vi "HFRR ADV v01.vi"() -> ()   [LabVIEW 2025] (continued)
            n3072 = case shown="True" w3184 {
              frame False {
              }
              frame True {
                n3073 = local write "Rt 3"(FALSE ("Rt 3")) -> ()
              }
            }
            "Rt" <- TRUE ("Rt")
            "Rt 2" <- FALSE ("Rt")
          }
          frame True {
            n3074 = local read "Rt"() -> (w3190:bool)
            n3075 = local write "Rt 2"(TRUE ("Rt 2")) -> ()
            n3076 = case shown="True" w3190 {
              frame False {
              }
              frame True {
                n3077 = local write "Rt"(FALSE ("Rt")) -> ()
              }
            }
            "Rt 3" <- TRUE ("Rt 3")
          }
        }
        n3078 = local read "Reset Graph"() -> (w3109:bool)
        n3079 = case shown="True" w3109 {
          selector: w3109 -> [_ w3133]
          frame False {
          }
          frame True {
            w3147 = 0.0 ("X Scale.Range:Maximum")
            n3080 = Not(x=w3133) -> (.not. x?=w3132:bool)
            n3081 = local write "Reset Graph"(w3132) -> ()
            n3082 = property on="Electrical Contact Resistance ( % )" class="WFChart (strict)"("XScale.Maximum"=600.0 ("X Scale.Range:Maximum"), "XScale.Minimum"=0.0 ("X Scale.Range:Minimum"), "YScale.Maximum"=100.0 ("Y Scale.Range:Maximum"), "YScale.Minimum"=0.0 ("Y Scale.Range:Minimum")) -> ()  [unwired: 2 in, 2 out]
            n3083 = property on="Frictional Force ( N )" class="WFChart (strict)"("XScale.Maximum"=600.0 ("X Scale.Range:Maximum"), "XScale.Minimum"=0.0 ("X Scale.Range:Minimum"), "YScale.Maximum"=100.0 ("Y Scale.Range:Maximum"), "YScale.Minimum"=0.0 ("Y Scale.Range:Minimum")) -> ()  [unwired: 2 in, 2 out]
            n3084 = property on="Temperature ( Deg C )" class="WFChart (strict)"("XScale.Maximum"=600.0 ("X Scale.Range:Maximum"), "XScale.Minimum"=0.0 ("X Scale.Range:Minimum"), "YScale.Maximum"=100.0 ("Y Scale.Range:Maximum"), "YScale.Minimum"=0.0 ("Y Scale.Range:Minimum")) -> ()  [unwired: 2 in, 2 out]
            n3085 = property on="Stroke ( mm )" class="WFChart (strict)"("XScale.Maximum"=600.0 ("X Scale.Range:Maximum"), "XScale.Minimum"=0.0 ("X Scale.Range:Minimum"), "YScale.Maximum"=100.0 ("Y Scale.Range:Maximum"), "YScale.Minimum"=0.0 ("Y Scale.Range:Minimum")) -> ()  [unwired: 2 in, 2 out]
            n3086 = property on="Coefficient of Friction" class="WFChart (strict)"("XScale.Maximum"=600.0 ("X Scale.Range:Maximum"), "XScale.Minimum"=0.0 ("X Scale.Range:Minimum"), "YScale.Maximum"=100.0 ("Y Scale.Range:Maximum"), "YScale.Minimum"=0.0 ("Y Scale.Range:Minimum")) -> ()  [unwired: 2 in, 2 out]
            n3087 = property on="Electrical Contact Resistance ( % )" class="WFChart (strict)"("XScale.Minimum"=0.0 ("X Scale.Range:Minimum"), "XScale.Maximum"=600.0 ("X Scale.Range:Maximum"), "YScale.Minimum"=0.0 ("Y Scale.Range:Minimum"), "YScale.Maximum"=100.0 ("Y Scale.Range:Maximum")) -> ()  [unwired: 2 in, 2 out]
            n3088 = property on="Temperature ( Deg C )" class="WFChart (strict)"("XScale.Minimum"=0.0 ("X Scale.Range:Minimum"), "XScale.Maximum"=600.0 ("X Scale.Range:Maximum"), "YScale.Minimum"=0.0 ("Y Scale.Range:Minimum"), "YScale.Maximum"=100.0 ("Y Scale.Range:Maximum")) -> ()  [unwired: 2 in, 2 out]
            n3089 = property on="Coefficient of Friction" class="WFChart (strict)"("XScale.Minimum"=0.0 ("X Scale.Range:Minimum"), "XScale.Maximum"=600.0 ("X Scale.Range:Maximum"), "YScale.Maximum"=1.0 ("X Scale.Range:Minimum"), "YScale.Minimum"=0.0 ("X Scale.Range:Minimum")) -> ()  [unwired: 2 in, 2 out]
            n3090 = property on="Frictional Force ( N )" class="WFChart (strict)"("XScale.Maximum"=600.0 ("X Scale.Range:Maximum"), "XScale.Minimum"=w3147, "YScale.Maximum"=10.0 ("Y Scale.Range:Maximum"), "YScale.Minimum"=w3147) -> ()  [unwired: 2 in, 2 out]
            n3091 = property on="Stroke ( mm )" class="WFChart (strict)"("XScale.Maximum"=600.0 ("X Scale.Range:Maximum"), "XScale.Minimum"=0.0 ("X Scale.Range:Minimum"), "YScale.Maximum"=100.0 ("Y Scale.Range:Maximum"), "YScale.Minimum"=0.0 ("Y Scale.Range:Minimum")) -> ()  [unwired: 2 in, 2 out]
          }
        }
      }
      frame "Compare Files" {
        # "Elapsed time\ncof\nstroke\nAir temp\nTemp\nHumidity"
        n3092 = case shown="True" "RSTV1 2" {
          frame False {
          }
          frame True {
            n3093 = property on="Humidity ( %RH )" class="XYGraph (strict)"("Y Scale.Display Format:Precision"=u8 0 ("Y Scale.Format & Precision:Precision")) -> ()  [unwired: 2 in, 2 out]
            n3094 = property on="Humidity ( %RH )" class="XYGraph (strict)"("X Scale.Range:Minimum"=0.0, "X Scale.Range:Maximum"=75.0, "Y Scale.Range:Minimum"=48.0, "Y Scale.Range:Maximum"=58.0) -> ()  [unwired: 2 in, 2 out]
          }
        }
        n3095 = case shown="True" "RST CP 2" {
          frame False {
          }
          frame True {
            n3096 = property on="XY Graph 13" class="XYGraph (strict)"("Y Scale.Display Format:Precision"=u8 0 ("Y Scale.Format & Precision:Precision")) -> ()  [unwired: 2 in, 2 out]
            n3097 = property on="XY Graph 13" class="XYGraph (strict)"("X Scale.Range:Minimum"=0.0, "X Scale.Range:Maximum"=75.0, "Y Scale.Range:Minimum"=0.0, "Y Scale.Range:Maximum"=100.0) -> ()  [unwired: 2 in, 2 out]
          }
        }
        n3098 = case shown="True" "RST CP" {
          frame False {
          }
          frame True {
            n3099 = property on="Sample Temperature ( °C )" class="XYGraph (strict)"("Y Scale.Display Format:Precision"=u8 2 ("Y Scale.Format & Precision:Precision")) -> ()  [unwired: 2 in, 2 out]
            n3100 = property on="Sample Temperature ( °C )" class="XYGraph (strict)"("X Scale.Range:Minimum"=0.0, "X Scale.Range:Maximum"=75.0, "Y Scale.Range:Minimum"=58.0, "Y Scale.Range:Maximum"=62.0) -> ()  [unwired: 2 in, 2 out]
          }
        }
        n3101 = case shown="True" "RSTV1 3" {
          frame False {
          }
          frame True {
            n3102 = property on="Air Temperature  ( °C )" class="XYGraph (strict)"("Y Scale.Display Format:Precision"=u8 2 ("Y Scale.Format & Precision:Precision")) -> ()  [unwired: 2 in, 2 out]
            n3103 = property on="Air Temperature  ( °C )" class="XYGraph (strict)"("X Scale.Range:Minimum"=0.0 ("Y Scale.Range:Minimum"), "X Scale.Range:Maximum"=75.0 ("Y Scale.Range:Maximum"), "Y Scale.Range:Minimum"=20.0 ("X Scale.Range:Minimum"), "Y Scale.Range:Maximum"=26.0 ("X Scale.Range:Maximum")) -> ()  [unwired: 2 in, 2 out]
          }
        }
        n3104 = case shown="True" "RSTV1 4" {
          frame False {
          }
          frame True {
            n3105 = property on="Stroke ( mm )" class="XYGraph (strict)"("Y Scale.Display Format:Precision"=u8 2 ("Y Scale.Format & Precision:Precision")) -> ()  [unwired: 2 in, 2 out]
            n3106 = property on="Stroke ( mm )" class="XYGraph (strict)"("X Scale.Range:Minimum"=0.0 ("Y Scale.Range:Maximum"), "X Scale.Range:Maximum"=75.0 ("X Scale.Range:Minimum"), "Y Scale.Range:Minimum"=0.98, "Y Scale.Range:Maximum"=1.02) -> ()  [unwired: 2 in, 2 out]
          }
        }
        n3107 = case shown="True" "rstv2" {
          frame False {
          }
          frame True {
            n3108 = property on="Coefficient Of Friction" class="XYGraph (strict)"("Y Scale.Display Format:Precision"=u8 3 ("Y Scale.Format & Precision:Precision")) -> ()  [unwired: 2 in, 2 out]
            n3109 = property on="Coefficient Of Friction" class="XYGraph (strict)"("X Scale.Range:Minimum"=0.0 ("Y Scale.Range:Maximum"), "X Scale.Range:Maximum"=75.0, "Y Scale.Range:Minimum"=0.0, "Y Scale.Range:Maximum"=1.0 ("X Scale.Range:Minimum")) -> ()  [unwired: 2 in, 2 out]
          }
        }
        n3110 = case shown="True" "RST CP 3" {
          frame False {
          }
          frame True {
            n3111 = property on="Air Temp ( °C ) vs Humidity ( % RH )" class="XYGraph (strict)"("X Scale.Range:Minimum"=18.0, "X Scale.Range:Maximum"=28.0 ("X Scale.Range:Minimum"), "Y Scale.Range:Minimum"=30.0 ("X Scale.Range:Minimum"), "Y Scale.Range:Maximum"=70.0 ("X Scale.Range:Minimum")) -> ()  [unwired: 2 in, 2 out]
          }
        }
        n3112 = case shown="True" "OPEN 1" {
          frame False {
          }
          frame True {
            (unwired) 0  # existing file
            w3900 = "Choose a datalog file to open"  # prompt
            n3113 = local write "OPEN 1"(FALSE ("OPEN 1")) -> ()
            n3114 = String To Path(string="C:\\LAB-IQ\\Data\\") -> (path=w3885:path)
            n3115 = File Dialog(6:"*.dgf" ("pattern"), 7:w3900, 11:w3885) -> (0:w3883:errorcluster, 3:w3891:path)  [unwired: 4 in, 2 out]
            n3116 = Unbundle(w3883) -> ()  [unwired: 3 out]
            n3117 = Strip Path(path=w3891) -> (name=w3890:string)  [unwired: 1 out]
            n3118 = Path To String(path=w3891) -> (string=w3886:string)
            "string1" <- w3886
            n3119 = Match Pattern(string=w3890, regular expression=".dgf") -> (before substring=→"String Control":string)  [unwired: 1 in, 3 out]
            n3120 = Match Pattern(string=w3886, regular expression=".dgf" ("substring (\"\")")) -> (before substring=w3896:string)  [unwired: 1 in, 3 out]
            n3121 = Concatenate Strings(w3896, ".duf" ("Substring")) -> (w3892:string)
            n3122 = String To Path(string=w3892) -> (path=w3897:path)
            n3123 = call <vilib>:"Read Characters From File.vi"("file path (dialog if empty)"=w3897, "start of read offset (chars.:0)"=60 ("start of read offset (chars.: 0)")) -> ("character string"=→"String Control 2":string)  [unwired: 4 in, 3 out]
          }
        }
        n3124 = case shown="True" "OPEN 2" {
          frame False {
          }
          frame True {
            (unwired) 0  # existing file
            w3918 = "Choose a datalog file to open"  # prompt
            n3125 = local write "OPEN 2"(FALSE ("OPEN 1")) -> ()
            n3126 = String To Path(string="C:\\LAB-IQ\\Data\\") -> (path=w3903:path)
            n3127 = File Dialog(6:"*.dgf" ("pattern"), 7:w3918, 11:w3903) -> (0:w3901:errorcluster, 3:w3909:path)  [unwired: 4 in, 2 out]
            n3128 = Unbundle(w3901) -> ()  [unwired: 3 out]
            n3129 = Strip Path(path=w3909) -> (name=w3907:string)  [unwired: 1 out]
            n3130 = Path To String(path=w3909) -> (string=w3904:string)
            "string1 2" <- w3904
            n3131 = Match Pattern(string=w3907, regular expression=".dgf") -> (before substring=→"String Control 3":string)  [unwired: 1 in, 3 out]
            n3132 = Match Pattern(string=w3904, regular expression=".dgf" ("substring (\"\")")) -> (before substring=w3915:string)  [unwired: 1 in, 3 out]
            n3133 = Concatenate Strings(w3915, ".duf" ("Substring")) -> (w3912:string)
            n3134 = String To Path(string=w3912) -> (path=w3910:path)
            n3135 = call <vilib>:"Read Characters From File.vi"("file path (dialog if empty)"=w3910, "start of read offset (chars.:0)"=60 ("start of read offset (chars.: 0)")) -> ("character string"=→"String Control 4":string)  [unwired: 4 in, 3 out]
          }
        }
        n3136 = case shown="True" "OPEN 3" {
          frame False {
          }
          frame True {
            (unwired) 0  # existing file
            w3936 = "Choose a datalog file to open"  # prompt
            n3137 = local write "OPEN 3"(FALSE ("OPEN 1")) -> ()
            n3138 = String To Path(string="C:\\LAB-IQ\\Data\\") -> (path=w3921:path)
            n3139 = File Dialog(6:"*.dgf" ("pattern"), 7:w3936, 11:w3921) -> (0:w3919:errorcluster, 3:w3927:path)  [unwired: 4 in, 2 out]
            n3140 = Unbundle(w3919) -> ()  [unwired: 3 out]
            n3141 = Strip Path(path=w3927) -> (name=w3925:string)  [unwired: 1 out]
            n3142 = Path To String(path=w3927) -> (string=w3922:string)
            "string1 3" <- w3922
            n3143 = Match Pattern(string=w3925, regular expression=".dgf") -> (before substring=→"String Control 5":string)  [unwired: 1 in, 3 out]
            n3144 = Match Pattern(string=w3922, regular expression=".dgf" ("substring (\"\")")) -> (before substring=w3932:string)  [unwired: 1 in, 3 out]
            n3145 = Concatenate Strings(w3932, ".duf" ("Substring")) -> (w3929:string)
            n3146 = String To Path(string=w3929) -> (path=w3933:path)
            n3147 = call <vilib>:"Read Characters From File.vi"("file path (dialog if empty)"=w3933, "start of read offset (chars.:0)"=60 ("start of read offset (chars.: 0)")) -> ("character string"=→"String Control 6":string)  [unwired: 4 in, 3 out]
          }
        }
        n3148 = case shown="True" "OPEN 4" {
          frame False {
          }
          frame True {
            (unwired) 0  # existing file
            w3954 = "Choose a datalog file to open"  # prompt
            n3149 = local write "OPEN 4"(FALSE ("OPEN 1")) -> ()
            n3150 = String To Path(string="C:\\LAB-IQ\\Data\\") -> (path=w3939:path)
            n3151 = File Dialog(6:"*.dgf" ("pattern"), 7:w3954, 11:w3939) -> (0:w3937:errorcluster, 3:w3945:path)  [unwired: 4 in, 2 out]
            n3152 = Unbundle(w3937) -> ()  [unwired: 3 out]
            n3153 = Strip Path(path=w3945) -> (name=w3943:string)  [unwired: 1 out]
            n3154 = Path To String(path=w3945) -> (string=w3940:string)
            "string1 4" <- w3940
            n3155 = Match Pattern(string=w3943, regular expression=".dgf") -> (before substring=→"String Control 7":string)  [unwired: 1 in, 3 out]
            n3156 = Match Pattern(string=w3940, regular expression=".dgf" ("substring (\"\")")) -> (before substring=w3950:string)  [unwired: 1 in, 3 out]
            n3157 = Concatenate Strings(w3950, ".duf" ("Substring")) -> (w3947:string)
            n3158 = String To Path(string=w3947) -> (path=w3951:path)
            n3159 = call <vilib>:"Read Characters From File.vi"("file path (dialog if empty)"=w3951, "start of read offset (chars.:0)"=60 ("start of read offset (chars.: 0)")) -> ("character string"=→"String Control 8":string)  [unwired: 4 in, 3 out]
          }
        }
      }
      frame "About" {
        # "Elapsed time\ncof\nstroke\nmean pos\nTemp\nHumidity"
        n3160 = disable-structure shown="Disabled" {
          frame Disabled {
            n3161 = case shown="True" "Export" {
              frame False {
              }
              frame True {
                w3976 = "                                      " ("string")
                w3978 = "\r"
                (unwired) i16 6 ("width (-)")
                w4055 = "\r"
                w3987 = "\r"
                n3162 = local write "Export"(FALSE ("Export")) -> ()
                n3163 = local read "String 29"() -> (w4024:string)
                n3164 = local read "String 34"() -> (w4012:string)
                n3165 = local read "String 35"() -> (w4007:string)
                n3166 = local read "String 37"() -> (w4003:string)
                n3167 = local read "String 36"() -> (w4000:string)
                n3168 = local read "String 38"() -> (w3997:string)
                n3169 = local read "String 39"() -> (w3994:string)
                n3170 = Match Pattern(string=w4024, regular expression=".dwm") -> (before substring=w4020:string)  [unwired: 1 in, 3 out]
                "before substring" <- w4020
                n3171 = local read "S 38"() -> (w4015:string)
                n3172 = local read "S 39"() -> (w4008:string)
                n3173 = local read "Temperature before test 2"() -> (w4044:dbl)
                n3174 = local read "Temperature after test 2"() -> (w4049:dbl)
                n3175 = local read "Humidity before test 2"() -> (w4030:dbl)
                n3176 = local read "Humidity after test 2"() -> (w4045:dbl)
                n3177 = local read "MWSD 2"() -> (w4041:dbl)
                n3178 = local read "WS1.4 2"() -> (w4057:dbl)
                n3179 = local read "HCF 2"() -> (w4053:dbl)
                n3180 = local read "AVP 2"() -> (w4042:dbl)
                n3181 = Concatenate Strings("1," ("string"), w4015) -> (w4014:string)
                n3182 = Concatenate Strings("2," ("string"), w4012) -> (w4011:string)
                n3183 = Concatenate Strings("3," ("string"), w4008) -> (w4010:string)
                n3184 = Concatenate Strings("4," ("string"), w4007) -> (w4006:string)
                n3185 = Concatenate Strings("5," ("string"), w4003) -> (w4004:string)
                n3186 = Concatenate Strings("6," ("string"), w4000) -> (w4001:string)
                n3187 = Concatenate Strings("7," ("string"), w3997) -> (w3998:string)
                n3188 = Concatenate Strings("8," ("string"), w3994) -> (w3995:string)
                n3189 = local read "Sample ID"() -> (w4062:string)
                n3190 = case shown="\"xlx\"" "Select File Type" {
                  tunnel: w4020 -> [w4065 w4067 w4069]
                  tunnel: [w4063 w4068 w4070] -> w4019
                  frame "xlx" {
                    n3191 = Concatenate Strings(w4065, ".xls" ("string")) -> (w4063:string)
                  }
                  frame "csv" {
                    n3192 = Concatenate Strings(w4067, ".csv" ("string")) -> (w4068:string)
                  }
                  frame "txt" {
                    n3193 = Concatenate Strings(w4069, ".txt" ("string")) -> (w4070:string)
                  }
                }
                n3194 = local read "Test Date"() -> (w4061:string)
                n3195 = local read "String 45"() -> (w3975:string)
                n3196 = local read "String 31"() -> (w4060:string)
                n3197 = local read "String 32"() -> (w4059:string)
                n3198 = local read "TITTLE"() -> (w3983:string)
                n3199 = Number To Fractional String(number=w4030, width (-)=i16 6, precision (6)=i16 2) -> (F-format string=w4029:string)  [unwired: 1 in]
                n3200 = Number To Fractional String(number=w4044, width (-)=i16 6, precision (6)=i16 2) -> (F-format string=w4050:string)  [unwired: 1 in]
                n3201 = Number To Fractional String(number=w4045, width (-)=i16 6, precision (6)=i16 2) -> (F-format string=w4043:string)  [unwired: 1 in]
                n3202 = Number To Fractional String(number=w4049, width (-)=i16 6, precision (6)=i16 2) -> (F-format string=w4048:string)  [unwired: 1 in]
                n3203 = Number To Fractional String(number=w4041, width (-)=i16 6, precision (6)=i16 2) -> (F-format string=w4039:string)  [unwired: 1 in]
                n3204 = Number To Fractional String(number=w4042, width (-)=i16 6, precision (6)=i16 2) -> (F-format string=w4040:string)  [unwired: 1 in]
                n3205 = Number To Fractional String(number=w4053, width (-)=i16 6, precision (6)=i16 2) -> (F-format string=w4054:string)  [unwired: 1 in]
                n3206 = Number To Fractional String(number=w4057, precision (6)=i16 2) -> (F-format string=w4058:string)  [unwired: 2 in]
                n3207 = local read "s.NO"() -> (w3977:string)
                n3208 = Concatenate Strings("=" ("string"), w3983) -> (w3982:string)
                n3209 = Concatenate Strings("S.No," ("string"), "                                       Parameters" ("string")) -> (w3988:string)
                n3210 = Concatenate Strings(w4055, w4014, w4029, w4055, w4011, w4050, w4055, w4010, w4043, w4055, w4006, w4048, w4055, w4004, w4039, w4055, w4001, w4040, w4055, w3998, w4054, w4055, w3995, w4058) -> (w4017:string)
                n3211 = Concatenate Strings(w3987, "," ("string"), w3975, w3977, w3976, w4059, w4062, w3976, w4060, w4061, w3987) -> (w3985:string)
                n3212 = local read "Tested by"() -> (w3991:string)
                n3213 = local read "String 33"() -> (w3992:string)
                n3214 = Concatenate Strings("," ("string"), "                                                                             " ("string")) -> (w3980:string)
                n3215 = Concatenate Strings(w3982, w3978, w3985, w3978, w3988, w4017, w3978, w3980, w3992, w3991) -> (→"export":string)
                n3216 = String To Path(string=w4019) -> (path=w4026:path)
                n3217 = local read "export"() -> (w4021:string)
                n3218 = call <vilib>:"Write Characters To File.vi"("append to file? (new file:F)"=FALSE, "character string"=w4021, "file path (dialog if empty)"=w4026) -> ()  [unwired: 2 in, 1 out]
              }
            }
          }
          frame Enabled {
          }
        }
        n3219 = case shown="True" "OK Button 17" {
          frame False {
          }
          frame True {
            (unwired) 0  # existing file
            w4279 = "Choose a datalog file to open"  # prompt
            n3220 = local write "OK Button 17"(FALSE ("OK Button 17")) -> ()
            n3221 = local read "String"() -> (w4274:string)
            n3222 = String To Path(string=w4274) -> (path=w4275:path)
            n3223 = File Dialog(6:"*.duf" ("pattern"), 7:w4279, 11:w4275) -> (0:w4266:errorcluster, 3:w4285:path)  [unwired: 4 in, 2 out]
            n3224 = Unbundle(w4266) -> ()  [unwired: 3 out]
            n3225 = Open/Create/Replace File "Open File"(file path (use dialog)=w4285) -> (refnum out=w4277:refnum<file>)  [unwired: 5 in, 2 out]
            n3226 = Strip Path(path=w4285) -> (name=w4283:string)  [unwired: 1 out]
            n3227 = Path To String(path=w4285) -> (string=w4268:string)
            n3228 = while {
              tunnel: w4277 -> [w4289]
              i -> [w4286]
              stop <- w4287 continue-if-true
              (unwired) TRUE ("line mode (F)")
              n3229 = Read from Text File "Read File"(file (use dialog)=w4289) -> (text=w4288:string)  [unwired: 3 in, 3 out]
              n3230 = local write "Numeric 16"(w4286) -> ()
              n3231 = String Length(string=w4288) -> (length=w4291:i32)
              n3232 = Greater?(x=w4291, y=1) -> (0:w4287:bool)
            }
            n3233 = local write "String 29"(w4268) -> ()
            n3234 = Search and Replace String(input string=w4268, search string=".duf", replace string=".dgf" ("replace string (\"\")")) -> (result string=→"String Indicator 4":string)  [unwired: 5 in, 3 out]
            n3235 = Match Pattern(string=w4283, regular expression=".dwm") -> (before substring=w4267:string)  [unwired: 1 in, 3 out]
            "String Indicator" <- w4267
            n3236 = Match Pattern(string=w4268, regular expression=".dwm" ("substring (\"\")")) -> (before substring=w4269:string)  [unwired: 1 in, 3 out]
            "String Indicator 3" <- w4269
            n3237 = local write "TITTLE 2"(w4267) -> ()
            n3238 = String To Path(string=w4269) -> (path=w4276:path)
            "path" <- w4276
            n3239 = call <vilib>:"Read Characters From File.vi"("file path (dialog if empty)"=w4276, "start of read offset (chars.:0)"=60 ("start of read offset (chars.: 0)")) -> ("character string"=→"String Indicator 2":string)  [unwired: 4 in, 3 out]
          }
        }
        n3240 = call <vilib>:"Query Available Printers.vi"() -> ("system configured printers"=w3968:string[])  [unwired: 9 in, 2 out]
        "System Configured Printers 2" <- w3968
        n3241 = local read "OK Button 16"() -> (w3965:bool)
        n3242 = case shown="True" "OK Button 16" {
          frame False {
          }
          frame True {
            n3243 = stacked-sequence {
              frame #0 {
                n3244 = local read "Numeric 16"() -> (w4293:i32)
                n3245 = local write "Numeric 10"(w4293) -> ()
              }
              frame #1 {
                n3246 = local read "String 29"() -> (w4296:string)
                n3247 = String To Path(string=w4296) -> (path=w4295:path)
                n3248 = Open/Create/Replace File "Open File"(file path (use dialog)=w4295) -> (refnum out=w4297:refnum<file>)  [unwired: 5 in, 2 out]
                n3249 = for {
                  N: 16 -> [_]
                  tunnel: w4297 -> [w4304]
                  i -> [w4300]
                  (unwired) TRUE ("line mode (F)")
                  n3250 = Read from Text File "Read File"(file (use dialog)=w4304) -> (text=w4298:string)  [unwired: 3 in, 3 out]
                  n3251 = Match Pattern(string=w4298, regular expression="(") -> (after substring=w4303:string)  [unwired: 1 in, 3 out]
                  n3252 = Match Pattern(string=w4303, regular expression=")") -> (before substring=w4299:string)  [unwired: 1 in, 3 out]
                  n3253 = case shown="1" w4300 {
                    tunnel: w4299 -> [w4305 w4306 _ _ w4307 w4308 w4309 w4311 w4313 w4315 w4317 w4319 w4321 w4323 _]
                    tunnel: w4298 -> [_ _ _ _ _ _ _ _ _ _ _ _ _ _ _]
                    frame 0 {
                      "TITTLE" <- w4305
                    }
                    frame 1 {
                      "Sample ID" <- w4306
                    }
                    frame 2 {
                    }
                    frame 3 {
                    }
                    frame 4 {
                      "Test Date" <- w4307
                    }
                    frame 5 {
                      "Tested by" <- w4308
                    }
                    frame 6 {
                      n3254 = Fract/Exp String To Number(string=w4309) -> (number=→"Humidity before test 2":dbl)  [unwired: 3 in, 1 out]
                    }
                    frame 7 {
                      n3255 = Fract/Exp String To Number(string=w4311) -> (number=→"Temperature before test 2":dbl)  [unwired: 3 in, 1 out]
                    }
                    frame 8 {
                      n3256 = Fract/Exp String To Number(string=w4313) -> (number=→"Humidity after test 2":dbl)  [unwired: 3 in, 1 out]
                    }
                    frame 9 {
                      n3257 = Fract/Exp String To Number(string=w4315) -> (number=→"Temperature after test 2":dbl)  [unwired: 3 in, 1 out]
                    }
                    frame 10 {
                      n3258 = Fract/Exp String To Number(string=w4317) -> (number=→"MWSD 2":dbl)  [unwired: 3 in, 1 out]
                    }
                    frame 11 {
                      n3259 = Fract/Exp String To Number(string=w4319) -> (number=→"AVP 2":dbl)  [unwired: 3 in, 1 out]
                    }
                    frame 12 {
                      n3260 = Fract/Exp String To Number(string=w4321) -> (number=→"HCF 2":dbl)  [unwired: 3 in, 1 out]
                    }
                    frame 13 {
                      n3261 = Fract/Exp String To Number(string=w4323) -> (number=→"WS1.4 2":dbl)  [unwired: 3 in, 1 out]
                    }
                    frame 14, Default {
                    }
                  }
                }
              }
              frame #2 {
              }
            }
            n3262 = local write "OK Button 16"(FALSE ("OK Button 13")) -> ()
          }
        }
        n3263 = Index Array(array=w3968, index="Select Printer 3") -> (element=w3970:string)
        "Selected Printer" <- w3970
        n3264 = case shown="True" w3965 {
          frame False {
          }
          frame True {
            n3265 = flat-sequence {
              frame #0 {
              }
              frame #1 {
                n3266 = Wait (ms)(milliseconds to wait=u32 100) -> ()  [unwired: 1 out]
              }
              frame #2 {
                n3267 = local write "OK Button 16"(FALSE ("Print 3")) -> ()
              }
            }
          }
        }
        n3268 = case shown="True" "Print" {
          tunnel: w3970 -> [_ w4262]
          frame False {
          }
          frame True {
            (unwired) i16 6 ("width (-)")
            (unwired) "TESTED BY : "
            (unwired) "TESTED DATE :"
            (unwired) "SAMPLE ID : "
            (unwired) "SAMPLE DESIGN : "
            w4220 = "\r"
            w4237 = "\r"
            # "add image"
            n3269 = local read "Sample ID"() -> (w4210:string)
            n3270 = local read "Tested by"() -> (w4213:string)
            n3271 = local read "String 34"() -> (w4200:string)
            n3272 = local read "String 45"() -> (w4180:string)
            n3273 = local read "String 35"() -> (w4195:string)
            n3274 = local read "String 37"() -> (w4193:string)
            n3275 = local read "String 32"() -> (w4215:string)
            n3276 = local read "String 36"() -> (w4190:string)
            n3277 = local read "String 31"() -> (w4214:string)
            n3278 = local read "Test Date"() -> (w4211:string)
            n3279 = local read "String 33"() -> (w4216:string)
            n3280 = local read "String 38"() -> (w4186:string)
            n3281 = local read "String 39"() -> (w4183:string)
            n3282 = local write "Print"(FALSE ("Print FF")) -> ()
            n3283 = local read "S 39"() -> (w4198:string)
            n3284 = local read "S 38"() -> (w4205:string)
            n3285 = local read "Temperature before test 2"() -> (w4236:dbl)
            n3286 = local read "Temperature after test 2"() -> (w4226:dbl)
            n3287 = local read "Humidity before test 2"() -> (w4251:dbl)
            n3288 = local read "Humidity after test 2"() -> (w4235:dbl)
            n3289 = local read "MWSD 2"() -> (w4240:dbl)
            n3290 = local read "WS1.4 2"() -> (w4218:dbl)
            n3291 = Concatenate Strings("2)" ("string"), w4200) -> (w4201:string)
            n3292 = Concatenate Strings("3)" ("string"), w4198) -> (w4199:string)
            n3293 = Concatenate Strings("1)" ("string"), w4205) -> (w4204:string)
            n3294 = Concatenate Strings("4)" ("string"), w4195) -> (w4196:string)
            n3295 = Concatenate Strings("5)" ("string"), w4193) -> (w4192:string)
            n3296 = Concatenate Strings("6)" ("string"), w4190) -> (w4189:string)
            n3297 = Concatenate Strings("7)" ("string"), w4186) -> (w4187:string)
            n3298 = Concatenate Strings("8)" ("string"), w4183) -> (w4184:string)
            n3299 = local read "HCF 2"() -> (w4222:dbl)
            n3300 = local read "AVP 2"() -> (w4239:dbl)
            n3301 = local read "s.NO"() -> (w4181:string)
            n3302 = call <vilib>:"New Report.vi"("report type"=enum16{"Standard Report", "HTML"}."Standard Report") -> ("report out"=w4260:refnum<class "NI_report.lvclass">, "error out"=w4259:errorcluster)  [unwired: 13 in]
            n3303 = local read "TITTLE"() -> (w4212:string)
            n3304 = Concatenate Strings(w4237, w4180, w4181, w4237, w4215, w4210, w4237, w4214, w4211, w4237, w4216, w4213, w4237) -> (w4230:string)
            "test by" <- w4230
            n3305 = Number To Fractional String(number=w4236, width (-)=i16 6, precision (6)=i16 2) -> (F-format string=w4225:string)  [unwired: 1 in]
            n3306 = Number To Fractional String(number=w4235, width (-)=i16 6, precision (6)=i16 2) -> (F-format string=w4238:string)  [unwired: 1 in]
            n3307 = Number To Fractional String(number=w4251, width (-)=i16 6, precision (6)=i16 2) -> (F-format string=w4256:string)  [unwired: 1 in]
            n3308 = Number To Fractional String(number=w4240, width (-)=i16 6, precision (6)=i16 2) -> (F-format string=w4242:string)  [unwired: 1 in]
            n3309 = Number To Fractional String(number=w4226, width (-)=i16 6, precision (6)=i16 2) -> (F-format string=w4227:string)  [unwired: 1 in]
            n3310 = Number To Fractional String(number=w4239, width (-)=i16 6, precision (6)=i16 2) -> (F-format string=w4241:string)  [unwired: 1 in]
            n3311 = Number To Fractional String(number=w4222, width (-)=i16 6, precision (6)=i16 2) -> (F-format string=w4221:string)  [unwired: 1 in]
            n3312 = Number To Fractional String(number=w4218, precision (6)=i16 2) -> (F-format string=w4217:string)  [unwired: 2 in]
            n3313 = call-dynamic "Set Report Header Text.vi"("report in"=w4260, "center header text"=w4212, "error in (no error)"=w4259) -> ("report out"=w4231:refnum<class "NI_report.lvclass">, "error out"=w4232:errorcluster)  [unwired: 11 in]
            n3314 = Concatenate Strings(w4220, w4204, w4256, w4220, w4201, w4225, w4220, w4199, w4238, w4220, w4196, w4227, w4220, w4192, w4242, w4220, w4189, w4241, w4220, w4187, w4221, w4220, w4184, w4217) -> (w4208:string)
            "export 2" <- w4208
            n3315 = call-poly <vilib>:"Append Report Text.vi"("report in"=w4231, "text"=w4230, "error in (no error)"=w4232) -> ("report out"=w4234:refnum<class "NI_report.lvclass">, "error out"=w4233:errorcluster)  [unwired: 9 in, 2 out]
            n3316 = local read "test by"() -> (w4207:string)
            n3317 = local read "TITTLE"() -> (w4209:string)
            n3318 = call-poly <vilib>:"Append Report Text.vi"("report in"=w4234, "error in (no error)"=w4233) -> ("report out"=w4255:refnum<class "NI_report.lvclass">, "error out"=w4253:errorcluster)  [unwired: 10 in, 2 out]
            n3319 = Concatenate Strings(w4209, w4208, w4207) -> (→"output":string)
            n3320 = call-poly <vilib>:"Append Report Text.vi"("report in"=w4255, "text"=w4208, "error in (no error)"=w4253) -> ("report out"=w4254:refnum<class "NI_report.lvclass">, "error out"=w4252:errorcluster)  [unwired: 9 in, 2 out]
            n3321 = call-dynamic "Print Report.vi"("report in"=w4254, "printer name (default)"=w4262, "error in (no error)"=w4252) -> ("report out"=w4264:refnum<class "NI_report.lvclass">, "error out"=w4265:errorcluster)  [unwired: 11 in]
            n3322 = call-dynamic "Dispose Report.vi"("report in"=w4264, "error in (no error)"=w4265) -> ()  [unwired: 13 in, 1 out]
          }
        }
        n3323 = case shown="True" "Print 2" {
          frame False {
          }
          frame True {
            n3324 = flat-sequence {
              frame #0 {
                n3325 = local read "s.NO"() -> (→"s.NO 2":string)
                n3326 = Wait (ms)(milliseconds to wait=u32 20) -> ()  [unwired: 1 out]
                n3327 = local read "Sample ID  3"() -> (→"Sample ID  6":string)
                n3328 = local read "Sample ID  4"() -> (→"Sample ID  7":string)
                n3329 = local read "Sample ID"() -> (→"Sample ID  2":string)
                n3330 = local read "Tested by"() -> (→"Tested by 2":string)
                n3331 = local read "Test Date"() -> (→"Test Date 2":string)
                n3332 = local read "Humidity after test 3"() -> (→"Humidity after test 4":dbl)
                n3333 = local read "Ref A Test Date :"() -> (→"TITTLE 4":string)
                n3334 = local read "Temperature before test 3"() -> (w4087:dbl)
                n3335 = local read "Temperature before test 3"() -> (→"Temperature after test 5":dbl)
                n3336 = local read "Temperature after test 3"() -> (→"Temperature after test 4":dbl)
                n3337 = local read "Humidity before test 3"() -> (→"Humidity before test 4":dbl)
                n3338 = local write "Temperature before test 3"(w4087) -> ()
                n3339 = local read "image data"() -> (w4078:T2)
                n3340 = String To Path(string="C:\\LAB-IQ\\im\\Temp_resized.jpg") -> (path=w4079:path)
                "path 2" <- w4079
                n3341 = call <vilib>:"Write JPEG File.vi"("image data"=w4078, "path to JPEG file"=w4079) -> ()  [unwired: 8 in, 2 out]
                "Ref A Test Date :" <- "Ref A Test Date :"
                "Ref B Test Date :" <- "Ref B Test Date :"
                "Ref B Scar Value :" <- "Ref B Scar Value :"
                "Ref A Scar Value :" <- "Ref A Scar Value :"
              }
              frame #1 {
                (unwired) HTML_Report_Image_Alignment."MIDDLE" ("alignment (default)")
                w4115 = u16 0 items=["portrait", "landscape"] ("orientation (portrait)")
                (unwired) HTML_Report_Image_Alignment."ABSMIDDLE" ("alignment (default)")
                (unwired) "TESTED BY : "
                (unwired) "TESTED DATE :"
                (unwired) "SAMPLE ID : "
                (unwired) "SAMPLE DESIGN : "
                w4148 = "\r"
                # "add image"
                n3342 = Wait (ms)(milliseconds to wait=u32 20) -> ()  [unwired: 1 out]
                n3343 = local read "Sample ID  2"() -> (w4141:string)
                n3344 = local read "Wear Scar X"() -> (w4113:dbl)
                "Length ( microns ) 2" <- w4113
                n3345 = local read "Wear Scar Y"() -> (w4112:dbl)
                "Wear Scar Y ( microns ) :" <- w4112
                n3346 = local read "Test Date 2"() -> (w4142:string)
                n3347 = local read "Tested by 2"() -> (w4143:string)
                n3348 = local read "String 46"() -> (w4139:string)
                n3349 = local read "String 48"() -> (w4145:string)
                n3350 = local read "String 47"() -> (w4144:string)
                n3351 = local read "String 49"() -> (w4146:string)
                n3352 = local read "String 10"() -> (w4099:string)
                n3353 = local read "s.NO 2"() -> (w4140:string)
                n3354 = Add(x=w4113, y=w4112) -> (x+y=w4111:dbl)
                n3355 = call <vilib>:"New Report.vi"("report type"=enum16{"Standard Report", "HTML"}."HTML") -> ("report out"=w4119:refnum<class "NI_report.lvclass">, "error out"=w4117:errorcluster)  [unwired: 13 in]
                n3356 = Concatenate Strings(w4148, w4139, w4140, w4148, w4145, w4141, w4148, w4144, w4142, w4148, w4146, w4143, w4148) -> (→"test by 2":string)
                n3357 = Concatenate Strings("C:\\LAB-IQ\\Data\\" ("string"), w4099, ".jpg" ("string")) -> ()  [unwired: 1 out]
                n3358 = Divide(x=w4111, y=2.0) -> (x/y=→"Mean Wear ( microns) :":dbl)
                n3359 = call-dynamic "Set Report Orientation.vi"("report in"=w4119, "orientation (portrait)"=w4115, "error in (no error)"=w4117) -> ("report out"=w4118:refnum<class "NI_report.lvclass">, "error out"=w4116:errorcluster)  [unwired: 11 in]
                n3360 = for {
                  N: 5 -> [_]
                  tunnel: w4118 -> [w4169]
                  tunnel: [w4168] -> w4097
                  tunnel: w4116 -> [w4167]
                  tunnel: [w4166] -> w4096
                  n3361 = call-dynamic "Set Report Tab Width.vi"("report in"=w4169, "error in (no error)"=w4167) -> ("report out"=w4168:refnum<class "NI_report.lvclass">, "error out"=w4166:errorcluster)  [unwired: 12 in]
                }
                n3362 = local read "TITTLE"() -> (w4114:string)
                n3363 = call-dynamic "Set Report Header Text.vi"("report in"=w4097, "center header text"=w4114, "error in (no error)"=w4096) -> ("report out"=w4135:refnum<class "NI_report.lvclass">, "error out"=w4134:errorcluster)  [unwired: 11 in]
                n3364 = for {
                  N: 1 -> [_]
                  tunnel: [w4173] -> w4121
                  tunnel: [w4172] -> w4120
                  tunnel: w4135 -> [w4171]
                  tunnel: w4134 -> [w4170]
                  n3365 = call-dynamic "New Report Line.vi"("report in"=w4171, "error in (no error)"=w4170) -> ("report out"=w4173:refnum<class "NI_report.lvclass">, "error out"=w4172:errorcluster)  [unwired: 12 in]
                }
                n3366 = for {
                  N: 2 -> [_]
                  tunnel: [w4165] -> w4127
                  tunnel: [w4164] -> w4126
                  tunnel: w4121 -> [w4163]
                  tunnel: w4120 -> [w4162]
                  n3367 = call-dynamic "New Report Line.vi"("report in"=w4163, "error in (no error)"=w4162) -> ("report out"=w4165:refnum<class "NI_report.lvclass">, "error out"=w4164:errorcluster)  [unwired: 12 in]
                }
                n3368 = for {
                  N: 25 -> [_]
                  tunnel: w4127 -> [w4161]
                  tunnel: w4126 -> [w4159]
                  tunnel: [w4160] -> w4130
                  tunnel: [w4158] -> w4129
                  n3369 = call-dynamic "Set Report Tab Width.vi"("report in"=w4161, "error in (no error)"=w4159) -> ("report out"=w4160:refnum<class "NI_report.lvclass">, "error out"=w4158:errorcluster)  [unwired: 12 in]
                }
                n3370 = control-ref of="Tab Control 9"() -> (w4125:refnum<vi>)
                n3371 = call-dynamic "Append Control Image to Report.vi"("report in"=w4130, "alignment (default)"=HTML_Report_Image_Alignment."ABSMIDDLE", "ctrl reference"=w4125, "error in (no error)"=w4129) -> ("report out"=w4124:refnum<class "NI_report.lvclass">, "error out"=w4123:errorcluster)  [unwired: 8 in, 2 out]
                n3372 = for {
                  N: 3 -> [_]
                  tunnel: [w4157] -> w4108
                  tunnel: [w4156] -> w4107
                  tunnel: w4124 -> [w4155]
                  tunnel: w4123 -> [w4154]
                  n3373 = call-dynamic "New Report Line.vi"("report in"=w4155, "error in (no error)"=w4154) -> ("report out"=w4157:refnum<class "NI_report.lvclass">, "error out"=w4156:errorcluster)  [unwired: 12 in]
                }
                n3374 = for {
                  N: 100 -> [_]
                  tunnel: w4108 -> [w4153]
                  tunnel: w4107 -> [w4151]
                  tunnel: [w4152] -> w4104
                  tunnel: [w4150] -> w4102
                  n3375 = call-dynamic "Set Report Tab Width.vi"("report in"=w4153, "error in (no error)"=w4151) -> ("report out"=w4152:refnum<class "NI_report.lvclass">, "error out"=w4150:errorcluster)  [unwired: 12 in]
                }
                n3376 = String To Path(string="C:\\LAB-IQ\\im\\Temp_resized.jpg") -> (path=w4094:path)
                n3377 = call-poly <vilib>:"Append Image to Report.vi"("report in"=w4104, "path or URL of image"=w4094, "error in (no error)"=w4102) -> ("report out"=w4103:refnum<class "NI_report.lvclass">, "error out"=w4101:errorcluster)  [unwired: 9 in, 2 out]
                n3378 = call-poly <vilib>:"Open HTML Report in Browser.vi"("report in"=w4103, "error in (no error)"=w4101) -> ("report out"=w4138:refnum<class "NI_report.lvclass">, "error out"=w4137:errorcluster)  [unwired: 11 in, 1 out]
                n3379 = call-dynamic "Dispose Report.vi"("report in"=w4138, "error in (no error)"=w4137) -> ()  [unwired: 13 in, 1 out]
              }
              frame #2 {
              }
              frame #3 {
                n3380 = disable-structure shown="Disabled" {
                  frame Disabled {
                    n3381 = local read "String 10"() -> (w4178:string)
                    n3382 = Concatenate Strings("C:\\LAB-IQ-NXT\\Data\\" ("string"), w4178, ".jpg" ("string")) -> (w4176:string)
                    n3383 = String To Path(string=w4176) -> (path=w4175:path)
                    n3384 = Delete(path (use dialog)=w4175) -> ()  [unwired: 4 in, 3 out]
                  }
                  frame Enabled {
                  }
                }
                n3385 = local write "Print 2"(FALSE ("Print")) -> ()
              }
            }
          }
        }
      }
    }
    n3386 = Wait (ms)(milliseconds to wait=u32 50) -> ()  [unwired: 1 out]
    n3387 = Wait (ms)(milliseconds to wait=u32 50) -> ()  [unwired: 1 out]
    n3388 = local read "Quit"() -> (w2401:bool)
  }
  n3389 = VISA Close(VISA resource name=w47, error in (no error)=w46) -> ()  [unwired: 1 out]
  n3390 = while {
    stop <- w4329 stop-if-true
    n3391 = local read "Auto Start Test"() -> (w4327:bool)
    n3392 = local read "RUN"() -> (w4326:bool)
    n3393 = Wait (ms)(milliseconds to wait=u32 1000) -> ()  [unwired: 1 out]
    n3394 = Or(x=w4326, y=w4327) -> (x .or. y?=w4325:bool)
    n3395 = case shown="True" w4325 {
      frame False {
      }
      frame True {
        n3396 = local read "LVDT STROKE Actual"() -> (w4330:dbl)
        n3397 = In Range and Coerce(upper limit=1.2, x=w4330, lower limit=0.6) -> (In Range?=w4333:bool)  [unwired: 1 out]
        n3398 = call-poly <vilib>:"Random Number (Range).vi"("lower bound (0)"=0.998 ("upper bound (100)"), "upper bound (100)"=1.003) -> ("number"=w4331:dbl)  [unwired: 9 in]
        n3399 = case shown="True" w4333 {
          tunnel: [w4338 w4339] -> w4332
          tunnel: w4331 -> [_ w4339]
          tunnel: w4330 -> [w4338 _]
          frame False {
          }
          frame True {
          }
        }
        "LVDT STROKE DISPLAY" <- w4332
      }
    }
    n3400 = local read "Quit"() -> (w4329:bool)
  }
  n3401 = while {
    tunnel: [w4356] -> w55
    shift-right: [w4349] -> _
    shift-left: 0.0 -> [w4352]
    shift-right: [w4348] -> _
    shift-left: 0.0 -> [w4351]
    shift-right: [w4347] -> _
    shift-left: 100.0 ("vc_cmd") -> [w4350]
    stop <- w4356 stop-if-true
    # "PID LOGIC"
    n3402 = local read "run test Calibration"() -> (w4344:bool)
    n3403 = local read "RUN"() -> (w4354:bool)
    n3404 = local read "Auto Start Temp"() -> (w4345:bool)
    n3405 = local read "Auto Start Test"() -> (w4353:bool)
    n3406 = local read "START TEMP"() -> (w4343:bool)
    n3407 = And(x=w4345, y=w4353) -> (x .and. y?=w4346:bool)
    n3408 = Or(x=w4354, y=w4346) -> (x .or. y?=w4355:bool)
    n3409 = And(x=w4355, y=w4343) -> (x .and. y?=w4342:bool)
    n3410 = And(x=w4344, y=w4343) -> (x .and. y?=w4341:bool)
    n3411 = Or(x=w4341, y=w4342) -> (x .or. y?=w4340:bool)
    n3412 = Wait (ms)(milliseconds to wait="milliseconds to wait") -> ()  [unwired: 1 out]
    n3413 = case shown="True" w4340 {
      tunnel: [400.0 ("out_vc_cmd") w4375] -> w4347
      tunnel: [w4359 w4377] -> w4348
      tunnel: [w4359 w4376] -> w4349
      tunnel: w4352 -> [_ w4366]
      tunnel: w4351 -> [_ w4365]
      tunnel: w4350 -> [_ w4364]
      tunnel: w4344 -> [_ w4360]
      frame False {
        w4359 = 0.0 ("error_out")
      }
      frame True {
        n3414 = case shown="True" w4360 {
          tunnel: [w4384 1.0] -> w4362
          frame False {
            n3415 = local read "Set Strk"() -> (w4383:dbl)
            n3416 = Add(x=w4383, y="Add up Stroke") -> (x+y=w4384:dbl)
          }
          frame True {
          }
        }
        n3417 = local read "LVDT STROKE"() -> (w4361:dbl)
        n3418 = formula code="// Zero-Hardcode Explicit Positional-Form PID Engine\n// Inputs: target_stroke, measured_stroke, dt, prev_error, integral_accumulator_in, prev_vc_cmd\n//         kp, ki, kd, max_step_change, max_amplitude, min_amplitude, startup_cmd\n// Outputs: vc_cmd, error_out, out_error, integral_accumulator_out, out_vc_cmd\n\n// 1. Calculate Tracking Error\nfloat current_error = target_stroke - measured_stroke;\nerror_out = current_error;\n\n// 2. Compute Proportional Term\nfloat p_term = kp * current_error;\n\n// 3. Compute Derivative Term\nfloat d_term = 0.0;\nif (dt > 0.0) {\n    d_term = kd * ((current_error - prev_error) / dt);\n}\n\n// 4. Update and Accumulate Integral Term\nfloat current_integral = integral_accumulator_in + (current_error * dt);\nfloat i_term = ki * current_integral;\n\n// 5. Calculate Ideal Target Command (Anchored by startup baseline)\nfloat ideal_command = startup_cmd + p_term + i_term + d_term;\n\n// 6. Apply Loop Rate Limiting FIRST \n// (Forces the command to climb gradually from prev_vc_cmd instead of jumping straight to max)\nfloat raw_adjustment = ideal_command - prev_vc_cmd;\n\nif (raw_adjustment > max_step_change) {\n    raw_adjustment = max_step_change;\n} else if (raw_adjustment < -max_step_change) {\n    raw_adjustment = -max_step_change;\n}\n\nfloat next_vc_cmd = prev_vc_cmd + raw_adjustment;\n\n// 7. Anti-Windup Protection & Final Output Safety Safeguard Clamping\n// (Back-calculating based on what we are ACTUALLY outputting)\nif (next_vc_cmd > max_amplitude) {\n    float excess = next_vc_cmd - max_amplitude;\n    if (ki > 0.0) {\n        current_integral -= excess / ki;\n    }\n    next_vc_cmd = max_amplitude;\n} else if (next_vc_cmd < min_amplitude) {\n    float excess = next_vc_cmd - min_amplitude;\n    if (ki > 0.0) {\n        current_integral -= excess / ki;\n    }\n    next_vc_cmd = min_amplitude;\n}\n\n// 8. Map to Shift Registers for memory persistence\nvc_cmd = next_vc_cmd;\nout_error = current_error;                   \nintegral_accumulator_out = current_integral;  \nout_vc_cmd = next_vc_cmd;"("target_stroke"=w4362, "measured_stroke"=w4361, "dt"="dt", "integral_accumulator_in"=w4365, "prev_error"=w4366, "prev_vc_cmd"=w4364, "kp"="kp", "ki"="ki", "kd"="kd", "max_step_change"="max_step_change", "max_amplitude"="max_amplitude", "min_amplitude"="min_amplitude", "startup_cmd"="startup_cmd") -> ("vc_cmd"=w4381:dbl, "out_error"=w4376:dbl, "integral_accumulator_out"=w4377:dbl, "out_vc_cmd"=w4375:dbl)  [unwired: 1 out]
        "output Vpp" <- w4381
        n3419 = Number To Fractional String(number=w4381, precision (6)=i16 1) -> (F-format string=w4379:string)  [unwired: 2 in]
        n3420 = Concatenate Strings("DAC;" ("string"), w4379) -> (w4363:string)
        n3421 = local write "Due Write"(w4363) -> ()
        "prev_error" <- w4366
        "integral_accumulator_in" <- w4365
        "prev_vc_cmd" <- w4364
      }
    }
    n3422 = local read "Quit"() -> (w4356:bool)
  }
  n3423 = Or(x=w51, y=w50) -> (x .or. y?=w52:bool)
  n3424 = Or(x=w48, y=w52) -> (x .or. y?=w57:bool)
  n3425 = control-ref of="new picture"() -> ()  [unwired: 1 out]
  n3426 = Or(x=w60, y=w57) -> (x .or. y?=w54:bool)
  n3427 = Or(x=w54, y=w55) -> (x .or. y?=w49:bool)
  n3428 = while {
    tunnel: [w4386] -> w59
    i -> [w4393]
    stop <- w4386 stop-if-true
    n3429 = local read "Quit"() -> (w4386:bool)
    n3430 = Equal To 0?(x=w4393) -> (x = 0?=w4391:bool)
    n3431 = call "Elapsed Time3"("Time Target (s)"=45.0, "Auto Reset"=TRUE) -> ("Time has Elapsed"=w4390:bool)  [unwired: 10 in, 7 out]
    n3432 = Wait (ms)(milliseconds to wait=u32 50) -> ()  [unwired: 1 out]
    n3433 = Or(x=w4390, y=w4391) -> (x .or. y?=w4392:bool)
    n3434 = case shown="True" w4392 {
      frame False {
      }
      frame True {
        n3435 = call <vilib>:"System Exec.vi"("run minimized? (F)"=TRUE, "error in (no error)"="error in (no error)", "command line"="powercfg.exe -change -monitor-timeout-ac 0") -> ("error out"=w4404:errorcluster)  [unwired: 5 in, 3 out]
        n3436 = call <vilib>:"System Exec.vi"("run minimized? (F)"=TRUE, "error in (no error)"=w4404, "command line"="powercfg.exe -change -disk-timeout-ac 0") -> ("error out"=w4403:errorcluster)  [unwired: 5 in, 3 out]
        n3437 = call <vilib>:"System Exec.vi"("run minimized? (F)"=TRUE, "error in (no error)"=w4403, "command line"="powercfg.exe -change -standby-timeout-ac 0") -> ("error out"=w4402:errorcluster)  [unwired: 5 in, 3 out]
        n3438 = call <vilib>:"System Exec.vi"("run minimized? (F)"=TRUE, "error in (no error)"=w4402, "command line"="powercfg.exe -change -hibernate-timeout-ac 0") -> ("error out"=w4401:errorcluster)  [unwired: 5 in, 3 out]
        n3439 = call <vilib>:"Simple Error Handler.vi"("error in (no error)"=w4401) -> ("error out"=w4407:errorcluster)  [unwired: 4 in, 4 out]
        n3440 = call <vilib>:"Clear Errors.vi"("error in (no error)"=w4407) -> ("error out"=→"error out":errorcluster)  [unwired: 5 in, 1 out]
      }
    }
  }
  n3441 = Compound Arithmetic op=OR(w62, w49, w59) -> (w61:bool)
  n3442 = flat-sequence {
    tunnel: w61 -> [_]
    tunnel: [w4409] -> w31
    tunnel: w31 -> [_]
    frame #0 {
      n3443 = call "CLOSE CONNECTION.vi"() -> ("error out"=w4409:errorcluster)  [unwired: 11 in]
    }
    frame #1 {
      n3444 = Quit LabVIEW(quit? (T)=TRUE) -> ()
      n3445 = local write "Quit"(FALSE ("EXIT")) -> ()
    }
  }
  n3446 = property on="Heater Button" class="Bool (strict)"("Visible"=TRUE) -> ()  [unwired: 2 in, 2 out]
  n3447 = while {
    tunnel: [w4416] -> _
    i -> [w4416]
    stop <- w4412 stop-if-true
    # "Langauage selection"
    n3448 = Equal?(x="Lan flag", y=22.0) -> ()  [unwired: 1 out]
    n3449 = disable-structure shown="Disabled" {
      frame Disabled {
        n3450 = stacked-sequence {
          frame #0 {
            n3451 = case shown="\"Russian\"" "Language Selection" {
              tunnel: [0 1] -> w4418
              frame "English", Default {
              }
              frame "Russian" {
              }
            }
            n3452 = for {
              N: 130 -> [_]
              tunnel: "Table" -> [w4427]
              tunnel: w4418 -> [w4426]
              i -> [w4425]
              n3453 = Index Array(array=w4427, index (row)=w4425, index (col)=w4426) -> (element=w4424:string)
              n3454 = case shown="4" w4425 {
                tunnel: w4424 -> [w4428 w4429 _ w4430 w4431 w4432 w4433 w4434 w4435 w4436 w4437 w4438 w4439 w4440 w4441 w4442 w4443 w4444 w4445 w4446 w4447 w4448 w4449 w4450 w4451 w4452 w4453 w4454 w4455 _ _ w4456 w4457 w4458 w4459 w4460 w4461 w4470 w4477 w4484 w4491 w4495 w4498 w4501 w4503 w4505 w4506 w4507 w4508 w4509 w4510 w4511 w4512 w4513 w4514 w4515 w4516 w4517 w4518 w4519 w4520 w4521 w4522 w4523 w4524 w4525 w4526 w4527 w4528 w4529 w4530 w4531 w4532 w4533 w4534 w4535 w4536 w4537 w4538 w4539 w4540 w4541 w4542 w4543 w4544 w4545 w4546 w4547 w4548 w4549 w4550 w4551 w4552 w4553 w4554 w4555 w4556 w4557 w4558 w4559 w4560 w4561 w4562 w4563 w4564 _ w4565 w4566 w4567 w4568 w4569 w4570 w4571 w4572 w4573 w4574 w4575 w4576 w4577 _ w4578 w4579 w4580 w4581 w4582 w4583 _]
                frame 0 {
                  n3455 = local write "S"(w4428) -> ()
                }
                frame 1 {
                  n3456 = local write "S 2"(w4429) -> ()
                }
                frame 2 {
                }
                frame 3 {
                  n3457 = local write "S 4"(w4430) -> ()
                }
                frame 4 {
                  n3458 = property on="FILE" class="Str"("Caption.Text"=w4431) -> ()  [unwired: 2 in, 2 out]
                }
                frame 5 {
                  n3459 = property on="Fuel Discription :" class="Str"("Caption.Text"=w4432) -> ()  [unwired: 2 in, 2 out]
                }
                frame 6 {
                  n3460 = property on="Remarks :" class="Str"("Caption.Text"=w4433) -> ()  [unwired: 2 in, 2 out]
                }
                frame 7 {
                  n3461 = property on="Save & Continue" class="Bool (strict)"("Boolean Text.Text"=w4434) -> ()  [unwired: 2 in, 2 out]
                }
                frame 8 {
                }
                frame 9 {
                  n3462 = property on="Set Hz" class="DigNum (strict)"("Caption.Text"=w4436) -> ()  [unwired: 2 in, 2 out]
                }
                frame 10 {
                }
                frame 11 {
                  n3463 = property on="NORMAL LOAD" class="DigNum (strict)"("Caption.Text"=w4438) -> ()  [unwired: 2 in, 2 out]
                }
                frame 12 {
                }
                frame 13 {
                  n3464 = property on="Set Temp" class="DigNum (strict)"("Caption.Text"=w4440) -> ()  [unwired: 2 in, 2 out]
                }
                frame 14 {
                  n3465 = local write "S 15"(w4441) -> ()
                }
                frame 15 {
                  n3466 = property on="Set Rh" class="DigNum (strict)"("Caption.Text"=w4442) -> ()  [unwired: 2 in, 2 out]
                }
                frame 16 {
                }
                frame 17 {
                  n3467 = local write "S 18"(w4444) -> ()
                }
                frame 18 {
                  "String 17" <- w4445
                }
                frame 19 {
                  n3468 = property on="test time" class="DigNum (strict)"("Caption.Text"=w4446) -> ()  [unwired: 2 in, 2 out]
                }
                frame 20 {
                  "String 18" <- w4447
                  "String 22" <- w4447
                }
                frame 21 {
                  n3469 = property on="Elapsed time" class="DigNum (strict)"("Caption.Text"=w4448) -> ()  [unwired: 2 in, 2 out]
                }
                frame 22 {
                  n3470 = property on="Samplingtime 2" class="DigNum (strict)"("Caption.Text"=w4449) -> ()  [unwired: 2 in, 2 out]
                }
                frame 23 {
                  "String 21" <- w4450
                }
                frame 24 {
                  n3471 = property on="Countdown" class="DigNum (strict)"("Caption.Text"=w4451) -> ()  [unwired: 2 in, 2 out]
                }
                frame 25 {
                  n3472 = property on="Countdown 2" class="DigNum (strict)"("Caption.Text"=w4452) -> ()  [unwired: 2 in, 2 out]
                }
                frame 26 {
                  n3473 = property on="Engage" class="Bool (strict)"("Boolean Text.Text"=w4453) -> ()  [unwired: 2 in, 2 out]
